vi "Handle Release Press.vi"(8 "error in (no error)":errorcluster, 11 "Stand in":refnum<class "Stand.lvclass">) -> (0 "error out":errorcluster, 3 "Stand out":refnum<class "Stand.lvclass">)   [LabVIEW 2019, in "Stand.lvclass"]
uses:
  Stand.lvclass
  D:/GIT H4000/H4000/src/Device_class/Device.lvclass
  Stand.lvclass/Stand.ctl
  TypeDef/handleModeState.ctl
  Device_class/Device.lvclass/Device.ctl
  FPGA/TypeDef/DO index.ctl
  AI_class/AI.lvclass/AI.ctl
  AnalogComparator_class/AnalogComparator.lvclass/AnalogComparator.ctl
  OscillationClass/OscillationDetector.lvclass/OscillationDetector.ctl
  TypeDef/Direction.ctl
  NeedleValve_class/NeedleValve.lvclass/NeedleValve.ctl
  TypeDef/Step_Name.ctl
  AI_class/Get_Values.vi
  AnalogComparator_class/GetStatus.vi
  NeedleValve_class/NeedleValve.lvclass
  FPGA_API_class/FPGA API.lvclass
  MessageInterface_class/MessageInterface.lvclass
  Device_class/Device.lvclass
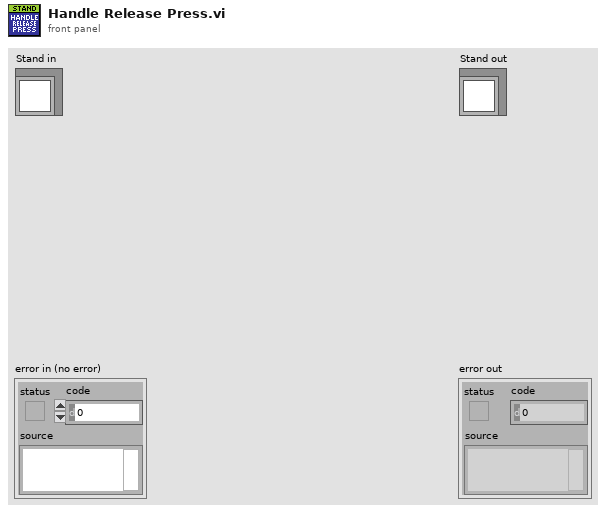
[diagram p1: front panel]
types:
  T1 = typedef "Step_Name.ctl" = enum16{"IDLE", "Filling", "Low Pressure", "Hi Pressure", "Abrupt Pressure Release", "Smooth Pressure Release", "Measuring Leakage Sensor 41.3", "Measuring Leakage Burette 42", "Alarm", "Stop Pump"}
  T2 = typedef "handleModeState.ctl" = enum16{"Init", "Run"}
  T3 = typedef "Direction.ctl" = enum16{"None", "DUT", "Chamber"}
  T4 = typedef "DO index.ctl" = u8
  T5 = typedef "Needle Valve Data.ctl" = cluster{"Engine State":T6, "StateValveModbus":T7, "Alarms":T8, "RAW":i32, "Angele":dbl, "Step":i32, "Encoder":i32, "Kinematic":T9, "Limits":T10, "EncoderMax":i32, "Counter Max Dont Update":i32, "EncoderMin":i32, "Counter Min Dont Update":i32, "Prepere Counter":i32, "STEP INIT":i32, "offset - Angel":dbl}
  T6 = typedef "MB_ENGINE.lvclass/Engine State.ctl" = u16
  T7 = typedef "Needle Valve State.ctl" = enum16{"STOPED", "CLOSED", "OPENED", "OPENING", "CLOSING"}
  T8 = typedef "MB_ENGINE.lvclass/Engine Alarms.ctl" = cluster{"OL":bool, "TF":bool, "STL":bool, "OCP":bool, "CPUV":bool, "UVLO":bool, "SPI_ERROR":bool, "Fault":bool, "OL 2":bool, "TF 2":bool, "STL 2":bool, "OCP 2":bool, "CPUV 2":bool, "UVLO 2":bool, "reserved":bool, "InitDone":bool}
  T9 = typedef "MB_ENGINE.lvclass/Settings.ctl" = cluster{"ACC Steps Per Sec^2":u16, "DEC Steps Per Sec^2":u16, "Min Velosity Step Per Sec":u16, "Max Velosity Step Per Sec":u16, "MicroStep":u16}
  T10 = typedef "MB_ENGINE.lvclass/Limits Status.ctl" = cluster{"Fault 2 Switch":bool, "Fault 1 Switch":bool, "Center(Home)":bool, "Lower Limit":bool, "Upper Limit":bool}
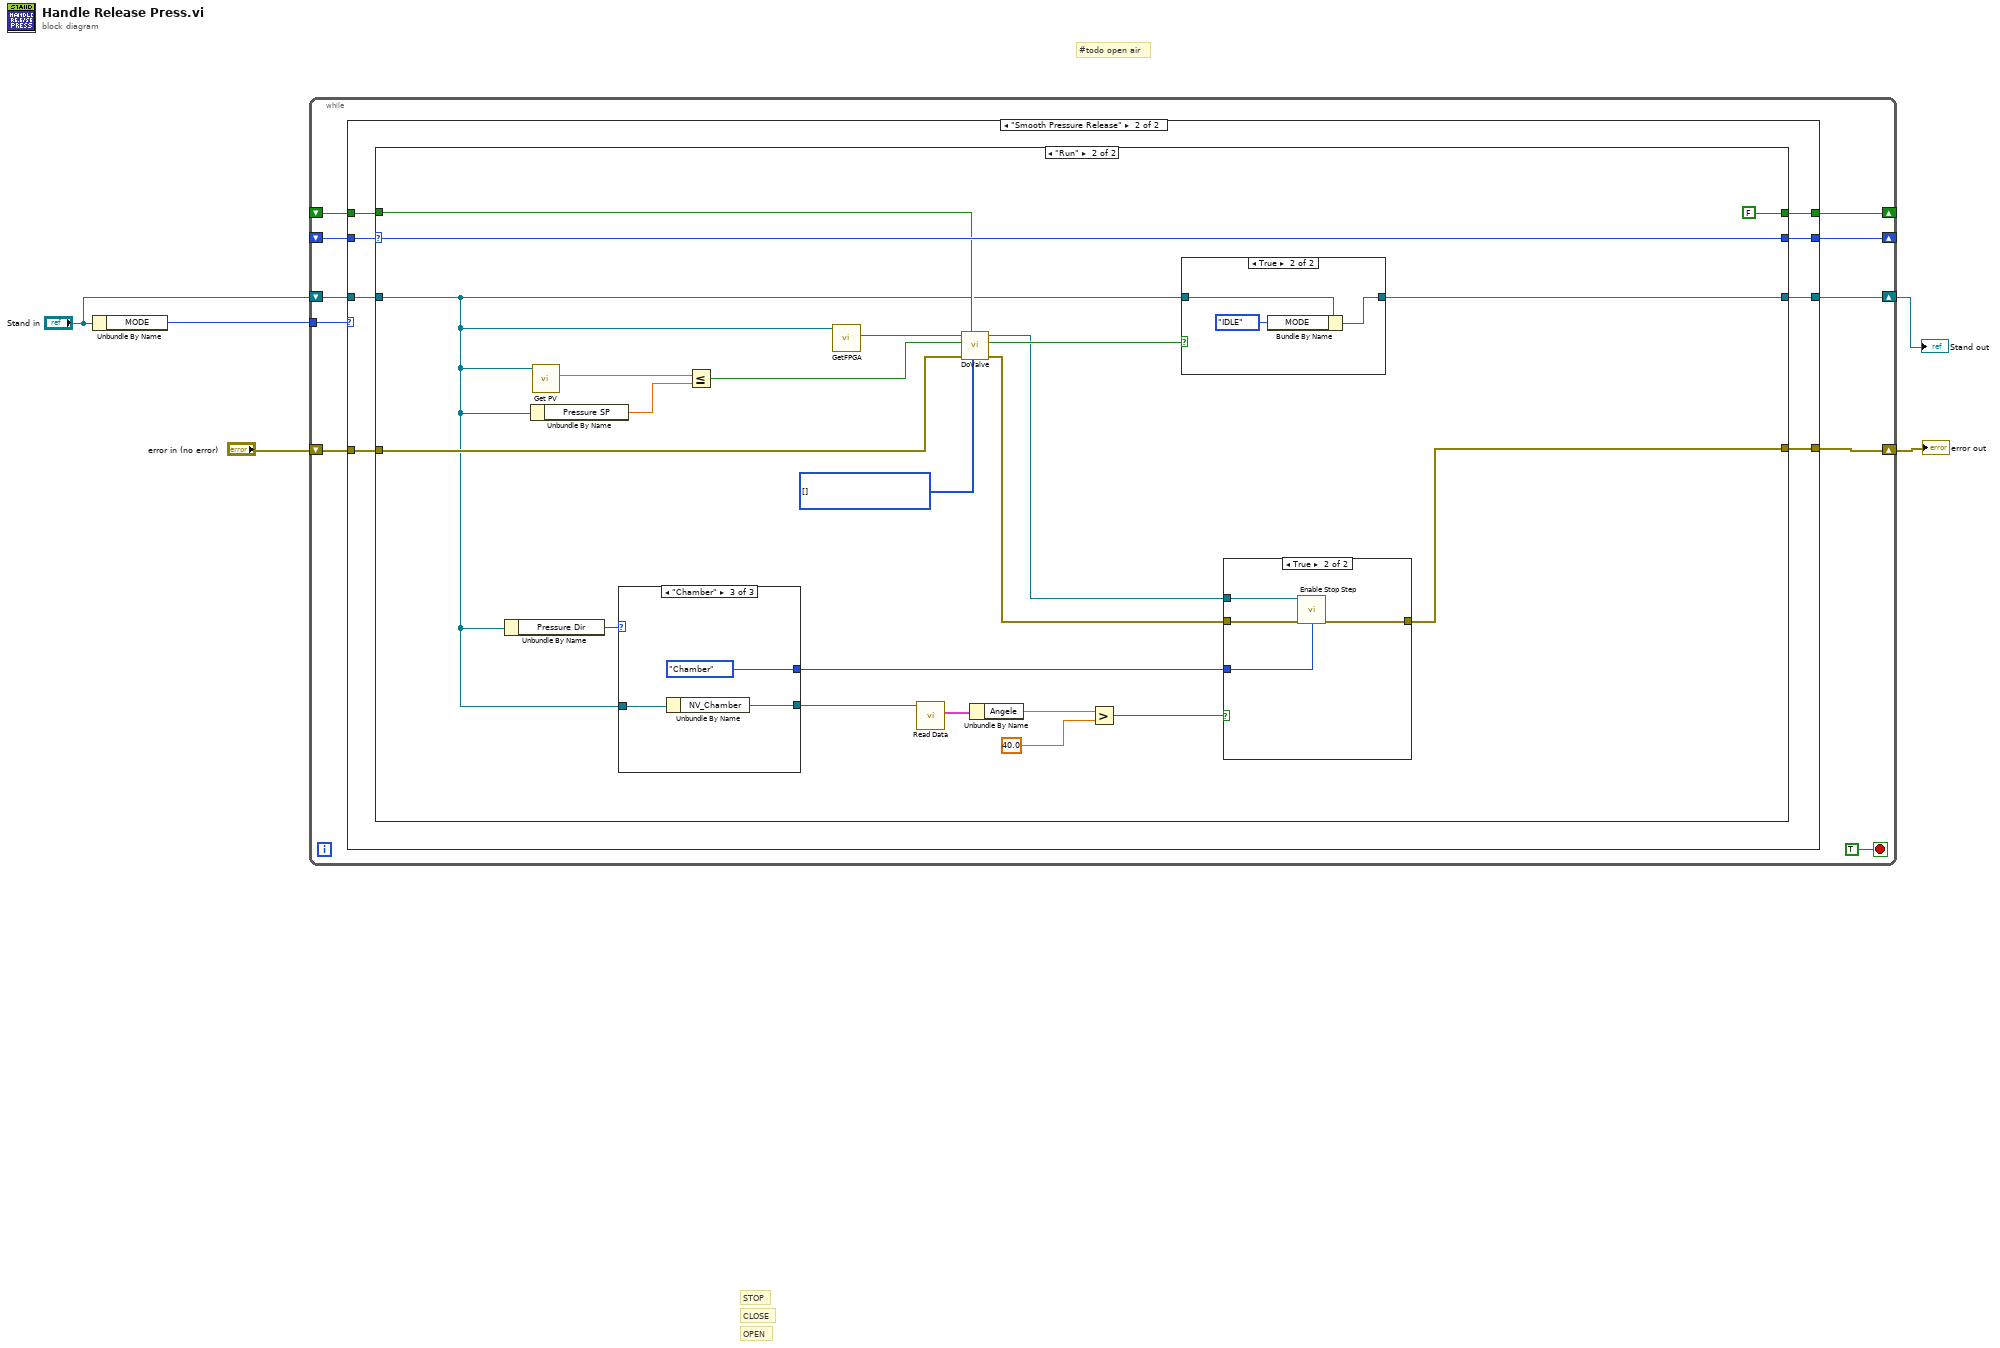
[diagram p0: block diagram]
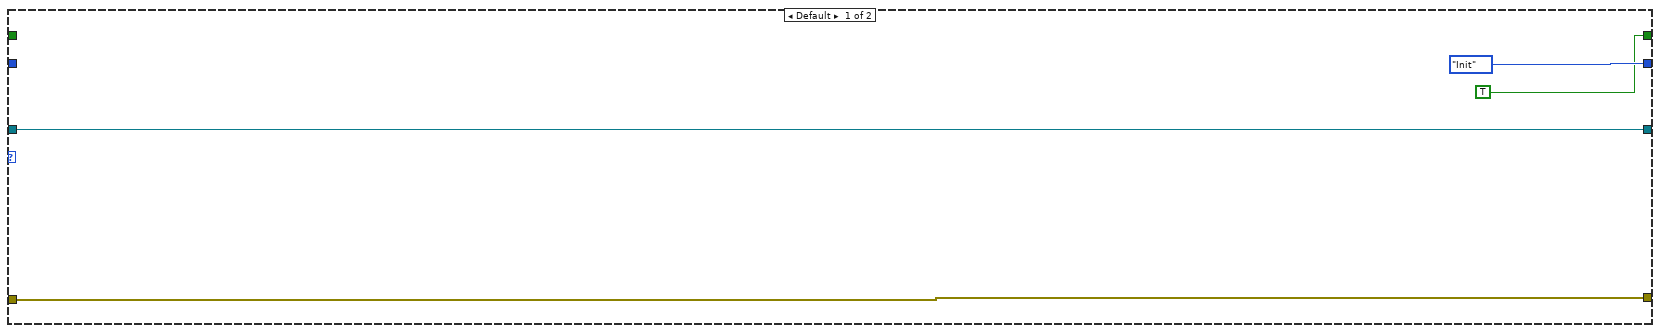
[diagram p2: hidden frame]
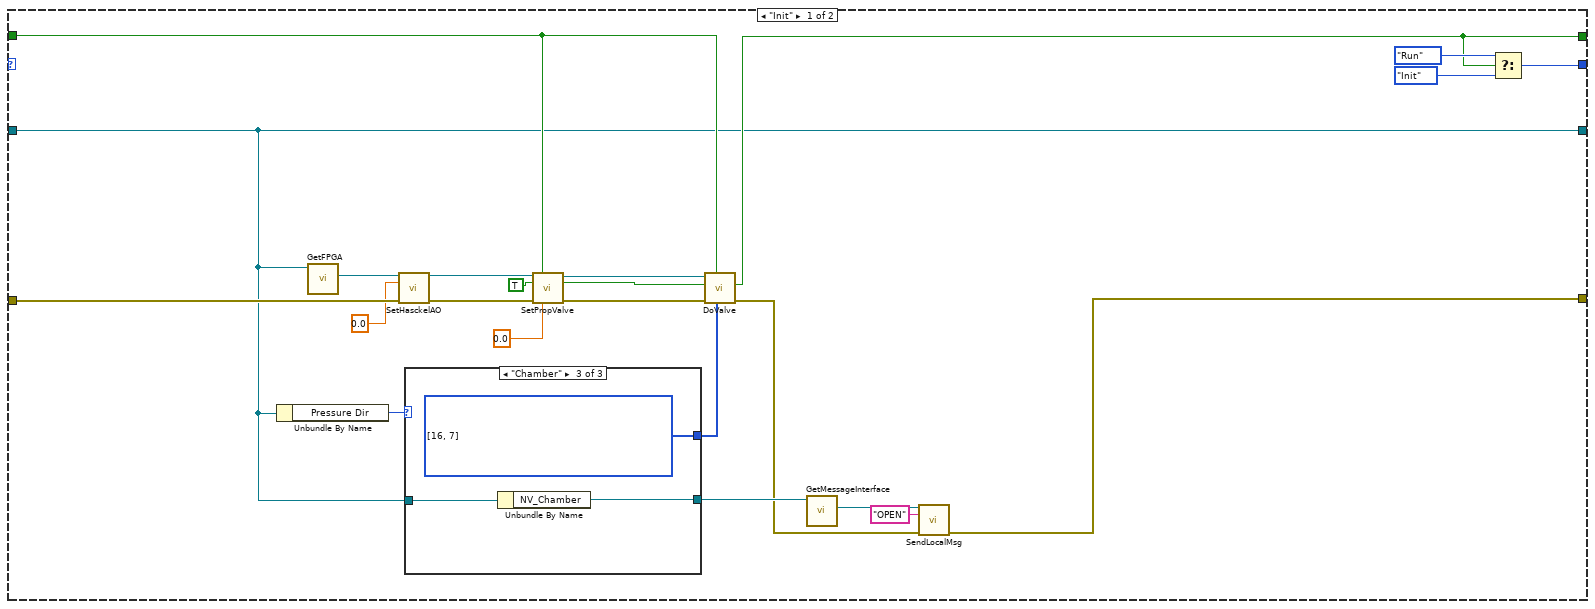
[diagram p3: hidden frame]
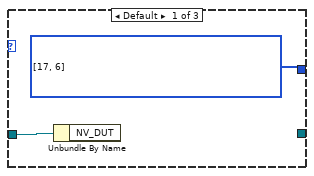
[diagram p4: hidden frame]
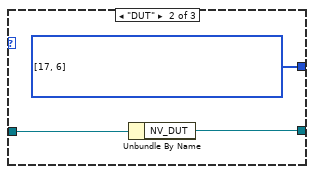
[diagram p5: hidden frame]
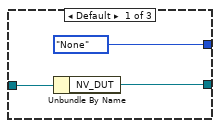
[diagram p6: hidden frame]
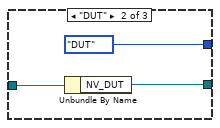
[diagram p7: hidden frame]
diagram:
  # "OPEN"
  # "CLOSE"
  # "STOP"
  # "#todo open air"
  n1 = Unbundle By Name("Stand in") -> ("MODE"=w2:T1)
  n2 = while {
    tunnel: w2 -> [w12]
    shift-right: [w15] -> w5
    shift-left: "error in (no error)" -> [w14]
    shift-right: [w11] -> w1
    shift-left: "Stand in" -> [w13]
    shift-right: [w9] -> _
    shift-left: _ -> [w8]
    shift-right: [w7] -> _
    shift-left: _ -> [w6]
    stop <- TRUE stop-if-true
    n3 = case shown="\"Smooth Pressure Release\"" w12 {
      tunnel: w14 -> [w19 w26]
      tunnel: [w19 w27] -> w15
      tunnel: w13 -> [w18 w25]
      tunnel: [w18 w24] -> w11
      tunnel: [handleModeState."Init" ("handleModeState") w20] -> w9
      tunnel: w8 -> [_ w23]
      tunnel: [TRUE w21] -> w7
      tunnel: w6 -> [_ w22]
      frame Default {
      }
      frame "Smooth Pressure Release" {
        n4 = case shown="\"Run\"" w23 {
          selector: w23 -> [_ w80]
          tunnel: [w30 w59] -> w27
          tunnel: w26 -> [w50 w71]
          tunnel: w25 -> [w28 w64]
          tunnel: [w28 w73] -> w24
          tunnel: w22 -> [w38 w74]
          tunnel: [w29 FALSE] -> w21
          tunnel: [w49 w80] -> w20
          frame "Init" {
            n5 = Unbundle By Name(w28) -> ("Pressure Dir"=w46:T3)
            n6 = call "GetFPGA.vi"("Device in"=w28) -> ("FPGA API.lvclass"=w44:refnum<class "FPGA API.lvclass">)  [unwired: 10 in]
            n7 = call-dynamic "SetHasckelAO.vi"("FPGA API in"=w44, "Haskel in"=0.0, "error in (no error)"=w50) -> ("FPGA API out"=w41:refnum<class "FPGA API.lvclass">, "error out"=w40:errorcluster)  [unwired: 11 in]
            n8 = case shown="\"Chamber\"" w46 {
              tunnel: [w52 w55 w58] -> w45
              tunnel: w28 -> [w51 w54 w57]
              tunnel: [_ w53 w56] -> w32
              frame Default {
                w52 = T4[] [17, 6] items=["DO 0 [KP1] [M12]", "DO 1 [ON KP2] [M21]", "DO 2 [ON KP3] [M24]", "DO 3 [WATER Y18.1 [DO3]]", "DO 4 [WATER Y18.2 [DO4]]", "DO 5 [KP6 Y29.1 33.7]", "DO 6 [KP7 Y29.2 33.8]", "DO 7 [KP8 Y29.3 33.9]", "DO 8 [KP9 Y29.4  33.12]", "DO 9 [KP10 Y29.5 33.1]", "DO 10 [KP11 Y29.6 33.2]", "DO 11 [KP12 Y29.7  33.13]", "DO 12 [KP13 Y29.8  33.11]", "DO 13 [KP14 Y29.9 33.10]", "DO 14 [KP15 Y29.10  33.6]", "DO 15 [KP16 Y29.11  33.5]", "DO 16 [KP17 Y29.12  33.4]", "DO 17 [KP18 Y29.13 33.3]", "DO 18 [AIR KP19]", "DO 19 [STEP DRIVE EN KP20]", "DO 20 [KP21 Y44.1 OPEN]", "DO 21 [ KP22 Y44.1 CLOSE]", "DO 22 [ KP23 Y44.2 OPEN]", "DO 23", "DO 24 [STEP DRIVE 1]", "DO 25 [STEP DRIVE 2]"] ("#DO")
                n9 = Unbundle By Name(w51) -> ()  [unwired: 1 out]
              }
              frame "DUT" {
                w55 = T4[] [17, 6] items=["DO 0 [KP1] [M12]", "DO 1 [ON KP2] [M21]", "DO 2 [ON KP3] [M24]", "DO 3 [WATER Y18.1 [DO3]]", "DO 4 [WATER Y18.2 [DO4]]", "DO 5 [KP6 Y29.1 33.7]", "DO 6 [KP7 Y29.2 33.8]", "DO 7 [KP8 Y29.3 33.9]", "DO 8 [KP9 Y29.4  33.12]", "DO 9 [KP10 Y29.5 33.1]", "DO 10 [KP11 Y29.6 33.2]", "DO 11 [KP12 Y29.7  33.13]", "DO 12 [KP13 Y29.8  33.11]", "DO 13 [KP14 Y29.9 33.10]", "DO 14 [KP15 Y29.10  33.6]", "DO 15 [KP16 Y29.11  33.5]", "DO 16 [KP17 Y29.12  33.4]", "DO 17 [KP18 Y29.13 33.3]", "DO 18 [AIR KP19]", "DO 19 [STEP DRIVE EN KP20]", "DO 20 [KP21 Y44.1 OPEN]", "DO 21 [ KP22 Y44.1 CLOSE]", "DO 22 [ KP23 Y44.2 OPEN]", "DO 23", "DO 24 [STEP DRIVE 1]", "DO 25 [STEP DRIVE 2]"] ("#DO")
                n10 = Unbundle By Name(w54) -> ("NV_DUT"=w53:refnum<class "NeedleValve.lvclass">)
              }
              frame "Chamber" {
                w58 = T4[] [16, 7] items=["DO 0 [KP1] [M12]", "DO 1 [ON KP2] [M21]", "DO 2 [ON KP3] [M24]", "DO 3 [WATER Y18.1 [DO3]]", "DO 4 [WATER Y18.2 [DO4]]", "DO 5 [KP6 Y29.1 33.7]", "DO 6 [KP7 Y29.2 33.8]", "DO 7 [KP8 Y29.3 33.9]", "DO 8 [KP9 Y29.4  33.12]", "DO 9 [KP10 Y29.5 33.1]", "DO 10 [KP11 Y29.6 33.2]", "DO 11 [KP12 Y29.7  33.13]", "DO 12 [KP13 Y29.8  33.11]", "DO 13 [KP14 Y29.9 33.10]", "DO 14 [KP15 Y29.10  33.6]", "DO 15 [KP16 Y29.11  33.5]", "DO 16 [KP17 Y29.12  33.4]", "DO 17 [KP18 Y29.13 33.3]", "DO 18 [AIR KP19]", "DO 19 [STEP DRIVE EN KP20]", "DO 20 [KP21 Y44.1 OPEN]", "DO 21 [ KP22 Y44.1 CLOSE]", "DO 22 [ KP23 Y44.2 OPEN]", "DO 23", "DO 24 [STEP DRIVE 1]", "DO 25 [STEP DRIVE 2]"] ("#DO")
                n11 = Unbundle By Name(w57) -> ("NV_Chamber"=w56:refnum<class "NeedleValve.lvclass">)
              }
            }
            n12 = call-dynamic "SetPropValve.vi"("FPGA API in"=w41, "Init"=w38, "Do"=TRUE, "error in (no error)"=w40, "AO 1"=0.0) -> ("FPGA API out"=w35:refnum<class "FPGA API.lvclass">, "Done"=w36:bool, "error out"=w39:errorcluster)  [unwired: 8 in]
            n13 = call "DoValve.vi"("#DO"=w45, "Init"=w38, "error in (no error)"=w39, "Do"=w36, "reference in"=w35) -> ("error out"=w31:errorcluster, "Done"=w29:bool)  [unwired: 4 in, 1 out]
            n14 = call "GetMessageInterface.vi"("Device in"=w32) -> ("MessageInterface"=w34:refnum<class "MessageInterface.lvclass">)  [unwired: 10 in]
            n15 = call-dynamic "SendLocalMsg.vi"("reference in"=w34, "name"="OPEN", "error in (no error)"=w31) -> ("error out"=w30:errorcluster)  [unwired: 10 in, 2 out]
            n16 = Select(t=handleModeState."Run", s=w29, f=handleModeState."Init") -> (s? t:f=w49:T2)
          }
          frame "Run" {
            w70 = T4[] [] items=["DO 0 [KP1] [M12]", "DO 1 [ON KP2] [M21]", "DO 2 [ON KP3] [M24]", "DO 3 [WATER Y18.1 [DO3]]", "DO 4 [WATER Y18.2 [DO4]]", "DO 5 [KP6 Y29.1 33.7]", "DO 6 [KP7 Y29.2 33.8]", "DO 7 [KP8 Y29.3 33.9]", "DO 8 [KP9 Y29.4  33.12]", "DO 9 [KP10 Y29.5 33.1]", "DO 10 [KP11 Y29.6 33.2]", "DO 11 [KP12 Y29.7  33.13]", "DO 12 [KP13 Y29.8  33.11]", "DO 13 [KP14 Y29.9 33.10]", "DO 14 [KP15 Y29.10  33.6]", "DO 15 [KP16 Y29.11  33.5]", "DO 16 [KP17 Y29.12  33.4]", "DO 17 [KP18 Y29.13 33.3]", "DO 18 [AIR KP19]", "DO 19 [STEP DRIVE EN KP20]", "DO 20 [KP21 Y44.1 OPEN]", "DO 21 [ KP22 Y44.1 CLOSE]", "DO 22 [ KP23 Y44.2 OPEN]", "DO 23", "DO 24 [STEP DRIVE 1]", "DO 25 [STEP DRIVE 2]"] ("#DO")
            n17 = Unbundle By Name(w64) -> ("Pressure Dir"=w65:T3)
            n18 = Unbundle By Name(w64) -> ("Pressure SP"=w76:dbl)
            n19 = call "Get PV.vi"("Stand in"=w64) -> ("Stat Data.scl mean"=w77:dbl)  [unwired: 10 in]
            n20 = case shown="\"Chamber\"" w65 {
              tunnel: w64 -> [w83 w86 w89]
              tunnel: [w82 w85 w88] -> w63
              tunnel: [Direction."None" ("Direction") Direction."DUT" ("Direction") Direction."Chamber" ("Direction")] -> w62
              frame Default {
                n21 = Unbundle By Name(w83) -> ("NV_DUT"=w82:refnum<class "NeedleValve.lvclass">)
              }
              frame "DUT" {
                n22 = Unbundle By Name(w86) -> ("NV_DUT"=w85:refnum<class "NeedleValve.lvclass">)
              }
              frame "Chamber" {
                n23 = Unbundle By Name(w89) -> ("NV_Chamber"=w88:refnum<class "NeedleValve.lvclass">)
              }
            }
            n24 = Less Or Equal?(x=w77, y=w76) -> (x <= y?=w75:bool)
            n25 = call "GetFPGA.vi"("Device in"=w64) -> ("FPGA API.lvclass"=w78:refnum<class "FPGA API.lvclass">)  [unwired: 10 in]
            n26 = call "Read Data.vi"("NeedleValve in"=w63) -> ("data value"=w69:T5)  [unwired: 10 in]
            n27 = call "DoValve.vi"("#DO"=w70, "Init"=w74, "error in (no error)"=w71, "Do"=w75, "reference in"=w78) -> ("error out"=w61:errorcluster, "Done"=w72:bool, "reference out"=w60:refnum<class "FPGA API.lvclass">)  [unwired: 4 in]
            n28 = Unbundle By Name(w69) -> ("Angele"=w68:dbl)
            n29 = Greater?(x=w68, y=40.0) -> (0:w66:bool)
            n30 = case shown="True" w72 {
              tunnel: w64 -> [w95 w98]
              tunnel: [w95 w97] -> w73
              frame False {
              }
              frame True {
                n31 = Bundle By Name(cluster=w98, "MODE"=Step_Name."IDLE" ("Data.MODE")) -> (w97:refnum<class "Stand.lvclass">)
              }
            }
            n32 = case shown="True" w66 {
              tunnel: [w90 w94] -> w59
              tunnel: w62 -> [_ w93]
              tunnel: w61 -> [w90 w92]
              tunnel: w60 -> [_ w91]
              frame False {
              }
              frame True {
                n33 = call-dynamic "Enable Stop Step.vi"("FPGA API in"=w91, "error in (no error)"=w92, "Direction"=w93) -> ("error out"=w94:errorcluster)  [unwired: 11 in, 1 out]
              }
            }
          }
        }
      }
    }
  }
  "error out" <- w5
  "Stand out" <- w1
